vi "ComputePoint.vi"(7 "Calibration":T2={"XHP ChirpGain"=1.0, "YHP ChirpGain"=1.0, "XLP ChirpGain"=1.0, "YLP ChirpGain"=1.0}, 8 "LP Center Frequency":u32=858993459 format="%x", 9 "HP Center Frequency":u32=805306367 format="%x", 10 "UpdatesPerPoint":u32, 11 "Point":cluster{"X":i32, "Y":i32, "Z":i32} {"Z" format="%x"; "Y" format="%x"; "X" format="%x"}) -> (3 "settings":T1 {"YLP_RR" format="%x"; "YLP_FR" format="%x"; "YHP_RR" format="%x"; "YHP_FR" format="%x"; "XLP_RR" format="%x"; "XLP_FR" format="%x"; "XHPstart" format="%x"; "XHPend" format="%x"; "XLPstart" format="%x"; "XLPend" format="%x"; "YHPstart" format="%x"; "YHPend" format="%x"; "YLPstart" format="%x"; "YLPend" format="%x"; "XHP_RR" format="%x"; "XHP_FR" format="%x"})   [LabVIEW 2012]
uses:
  AODCalibration.ctl
  CoordinateSettings.ctl
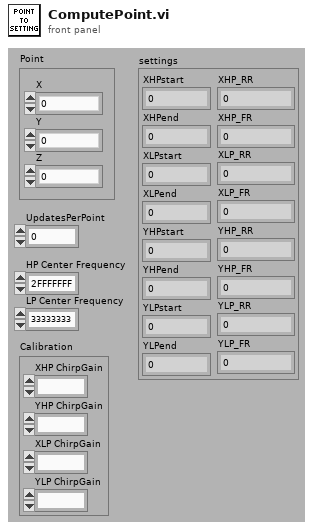
[diagram p1: front panel]
types:
  T1 = typedef "CoordinateSettings.ctl" = cluster{"XHPstart":u32, "XHPend":u32, "XLPstart":u32, "XLPend":u32, "YHPstart":u32, "YHPend":u32, "YLPstart":u32, "YLPend":u32, "XHP_RR":u32, "XHP_FR":u32, "XLP_FR":u32, "XLP_RR":u32, "YHP_FR":u32, "YHP_RR":u32, "YLP_FR":u32, "YLP_RR":u32}
  T2 = typedef "AODCalibration.ctl" = cluster{"XHP ChirpGain":fxp<+/-,16,2>, "YHP ChirpGain":fxp<+/-,16,2>, "XLP ChirpGain":fxp<+/-,16,2>, "YLP ChirpGain":fxp<+/-,16,2>}
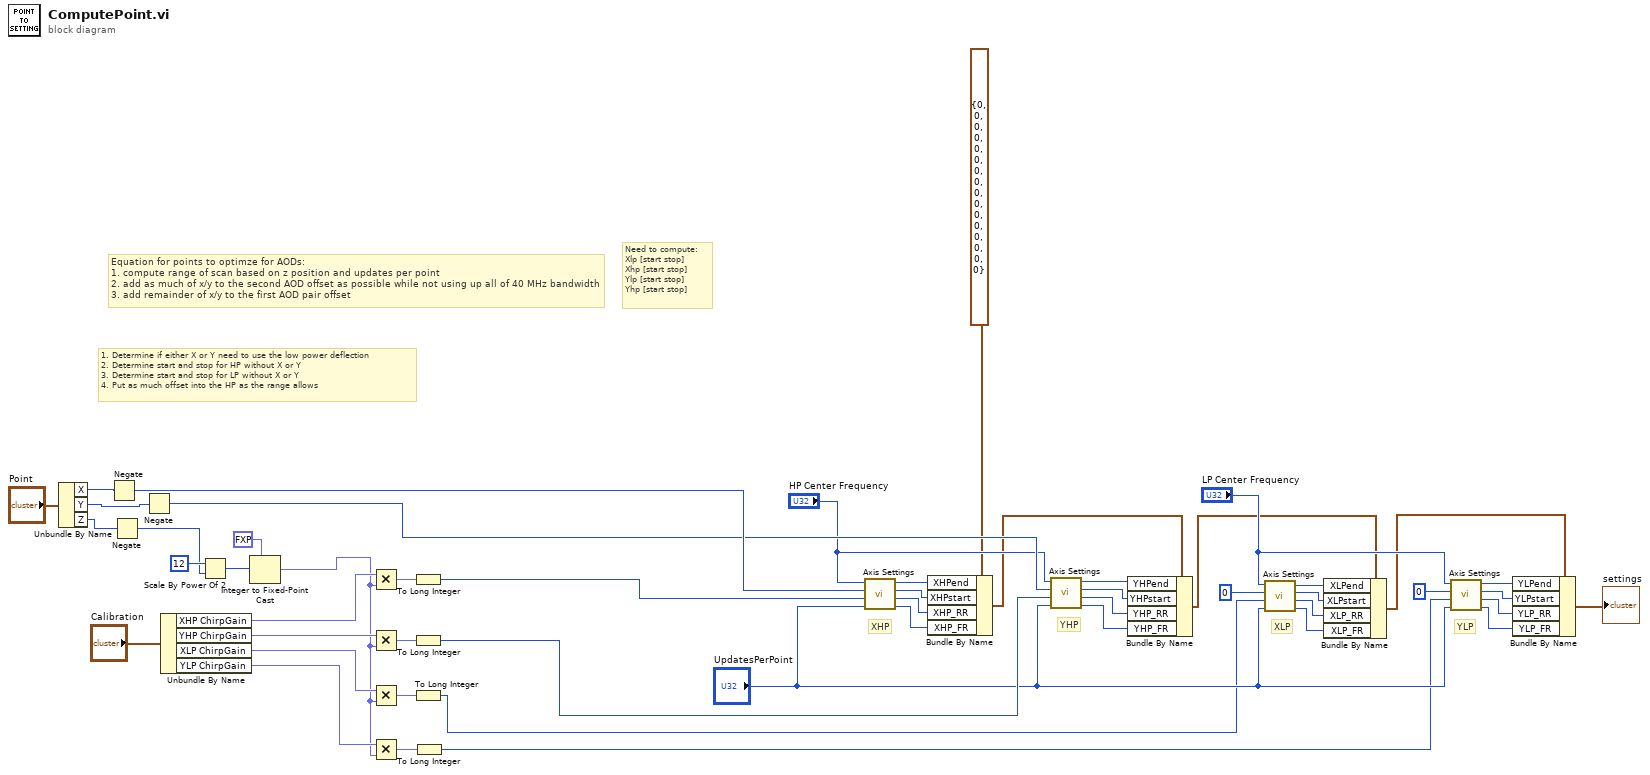
[diagram p0: block diagram]
diagram:
  # "YLP"
  # "XLP"
  # "YHP"
  # "XHP"
  # "1. Determine if either X or Y need to use the low power deflection\n2. Determine start and stop for HP without X or Y\n3. Determine start and stop for LP without X or Y\n4. Put as much offset into the HP as the range allows"
  # "Need to compute:\nXlp [start stop]\nXhp [start stop]\nYlp [start stop]\nYhp [start stop]"
  # "Equation for points to optimze for AODs:\n1. compute range of scan based on z position and updates per point\n2. add as much of x/y to the second AOD offset as possible while not using up all of 40 MHz bandwidth\n3. add remainder of x/y to the first AOD pair offset"
  n1 = Unbundle By Name("Point") -> ("X"=w49:i32, "Y"=w48:i32, "Z"=w47:i32)
  n2 = Negate(x=w49) -> (-x=w37:i32)
  n3 = Negate(x=w47) -> (-x=w1:i32)
  n4 = Negate(x=w48) -> (-x=w36:i32)
  n5 = Unbundle By Name("Calibration") -> ("XHP ChirpGain"=w45:fxp<+/-,16,2>, "YHP ChirpGain"=w44:fxp<+/-,16,2>, "XLP ChirpGain"=w43:fxp<+/-,16,2>, "YLP ChirpGain"=w42:fxp<+/-,16,2>)
  n6 = Scale By Power Of 2(n=12, x=w1) -> (x*2^n=w4:i32)
  n7 = Integer to Fixed-Point Cast(fixed-point type=fxp<+/-,32,20> 0.0, integer=w4) -> (fixed-point=w3:fxp<+/-,32,20>)
  n8 = Multiply(x=w45, y=w3) -> (x*y=w41:fxp<+/-,48,22>)
  n9 = Multiply(x=w44, y=w3) -> (x*y=w40:fxp<+/-,48,22>)
  n10 = Multiply(x=w43, y=w3) -> (x*y=w39:fxp<+/-,48,22>)
  n11 = Multiply(x=w42, y=w3) -> (x*y=w38:fxp<+/-,48,22>)
  n12 = To Long Integer(number=w41) -> (32bit integer=w29:i32)
  n13 = To Long Integer(number=w40) -> (32bit integer=w28:i32)
  n14 = To Long Integer(number=w39) -> (32bit integer=w24:i32)
  n15 = To Long Integer(number=w38) -> (32bit integer=w22:i32)
  n16 = call "Axis Settings.vi"("Updates Per Point"="UpdatesPerPoint", "Ramp"=w29, "Offset"=w37, "Center Frequency"="HP Center Frequency") -> ("Falling Rate"=w30:u32, "Rising Rate"=w31:u32, "Low"=w32:u32, "High"=w33:u32)  [unwired: 4 in]
  n17 = Bundle By Name(cluster=T1 {"XHPstart"=0, "XHPend"=0, "XLPstart"=0, "XLPend"=0, "YHPstart"=0, "YHPend"=0, "YLPstart"=0, "YLPend"=0, "XHP_RR"=0, "XHP_FR"=0, "XLP_FR"=0, "XLP_RR"=0, "YHP_FR"=0, "YHP_RR"=0, "YLP_FR"=0, "YLP_RR"=0} ("settings"), "XHPend"=w33, "XHPstart"=w32, "XHP_RR"=w31, "XHP_FR"=w30) -> (w17:T1)
  n18 = call "Axis Settings.vi"("Updates Per Point"="UpdatesPerPoint", "Ramp"=w28, "Offset"=w36, "Center Frequency"="HP Center Frequency") -> ("Falling Rate"=w18:u32, "Rising Rate"=w19:u32, "Low"=w20:u32, "High"=w21:u32)  [unwired: 4 in]
  n19 = Bundle By Name(cluster=w17, "YHPend"=w21, "YHPstart"=w20, "YHP_RR"=w19, "YHP_FR"=w18) -> (w16:T1)
  n20 = call "Axis Settings.vi"("Updates Per Point"="UpdatesPerPoint", "Ramp"=w24, "Offset"=0, "Center Frequency"="LP Center Frequency") -> ("Falling Rate"=w12:u32, "Rising Rate"=w13:u32, "Low"=w14:u32, "High"=w15:u32)  [unwired: 4 in]
  n21 = Bundle By Name(cluster=w16, "XLPend"=w15, "XLPstart"=w14, "XLP_RR"=w13, "XLP_FR"=w12) -> (w11:T1)
  n22 = call "Axis Settings.vi"("Updates Per Point"="UpdatesPerPoint", "Ramp"=w22, "Offset"=0, "Center Frequency"="LP Center Frequency") -> ("Falling Rate"=w7:u32, "Rising Rate"=w8:u32, "Low"=w9:u32, "High"=w10:u32)  [unwired: 4 in]
  n23 = Bundle By Name(cluster=w11, "YLPend"=w10, "YLPstart"=w9, "YLP_RR"=w8, "YLP_FR"=w7) -> (→"settings":T1)
